vi "Read iaa.vi"(8 "error in (no error)":errorcluster, 11 "IAA.lvclass in":refnum<class "IAA.lvclass">) -> (0 "error out":errorcluster, 2 "iaa":dbl[unit] min=-6.283185307179586 max=6.283185307179586, 3 "IAA.lvclass out":refnum<class "IAA.lvclass">)   [LabVIEW 2009, in "IAA.lvclass"]
uses:
  IAA.lvclass
  IAA.lvclass/IAA.ctl
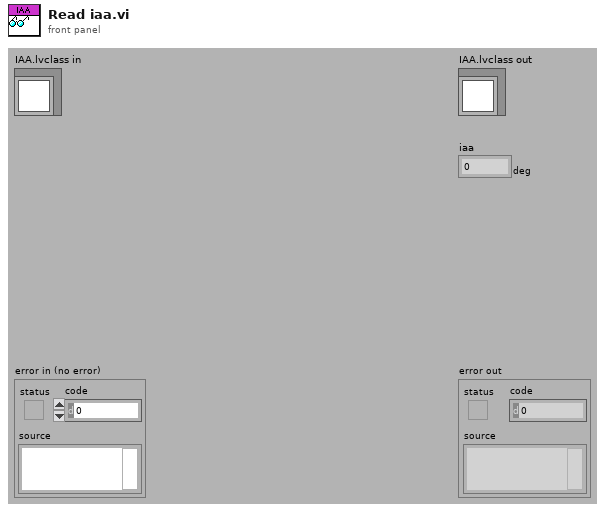
[diagram p1: front panel]
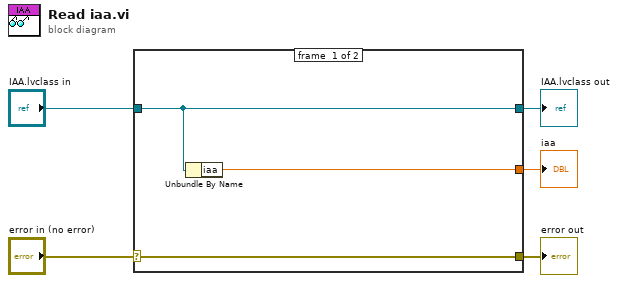
[diagram p0: block diagram]
diagram:
  n1 = case shown="No Error" "error in (no error)" {
    selector: "error in (no error)" -> [w8 w9]
    tunnel: [w8 w9] -> w4
    tunnel: [w7 w10] -> w2
    tunnel: "IAA.lvclass in" -> [w7 w10]
    tunnel: [w6 _] -> w1
    frame #0 {
      n2 = Unbundle By Name(w7) -> ("iaa"=w6:dbl[unit])
    }
    frame #1 {
    }
  }
  "error out" <- w4
  "IAA.lvclass out" <- w2
  "iaa" <- w1
